vi "makeFitPlotCommands.vi"(5 "Fit Zmin":dbl=500.0 min=0.0, 6 "plotInfoArray":T1(array[cluster]), 7 "Fit Zmax":dbl=500.0 min=0.0, 9 "BL Targets":T2[](array[typedef]) {"n" min=0.02 max=0.5 step=0.01 format="%.2f"}, 10 "Coefficients":cluster{"No d0":T3, "with d0":T3}, 11 "Zref":dbl=508.0 min=0.0) -> (1 "UnderlayPlotSeries":string[](array[string])=["fitmin = 100, fitmax=550, zref=508, d=16.2, n=0.121, clippedpowerlaw(x) w line ls 1 lw 10 lc rgb \"gray25\" title 'fit with displacement'", "fitmin = 100, fitmax=550, zref=508, d=0, n=0.133, clippedpowerlaw(x) w line ls 1 lw 8 lc rgb \"gray50\" title 'zero displacement fit'", "zref=508, d=0, n=0.170, powerlaw(x) w line ls 0 lw 1 lc rgb \"gray75\" title 'target power law'"], 2 "Pre-plot Injection":string, 3 "BasicsVisible":bool[](array[boolean]))   [LabVIEW 2021]
uses:
  PowerLaw.ctl
  BLTarget.ctl
  at.ctl
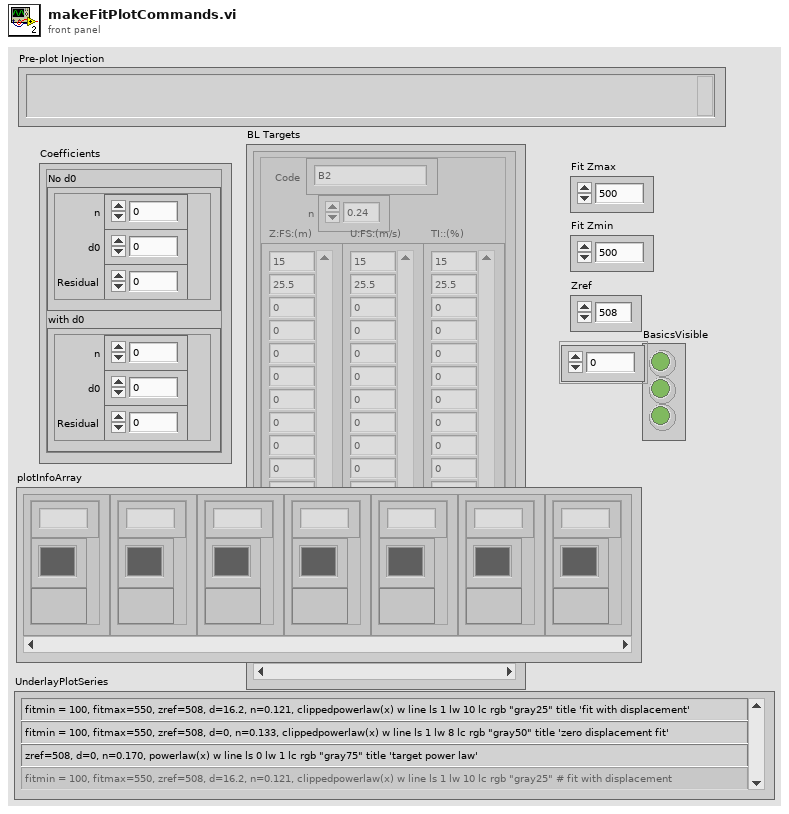
[diagram p1: front panel]
types:
  T1 = cluster{"Plot Name":string, "Plot.Plot Color":u32, "Plot.Visible?":bool}[]
  T2 = typedef "BLTarget.ctl" = cluster{"Code":string, "n":dbl, "Z:FS:(m)":dbl[], "U:FS:(m/s)":dbl[], "TI::(%)":dbl[]}
  T3 = typedef "PowerLaw.ctl" = cluster{"n":dbl, "d0":dbl, "Residual":dbl}
  T4 = typedef "at.ctl" = cluster{"XcoordSys":string, "YcoordSys":string, "Xvalue":dbl, "Yvalue":dbl}
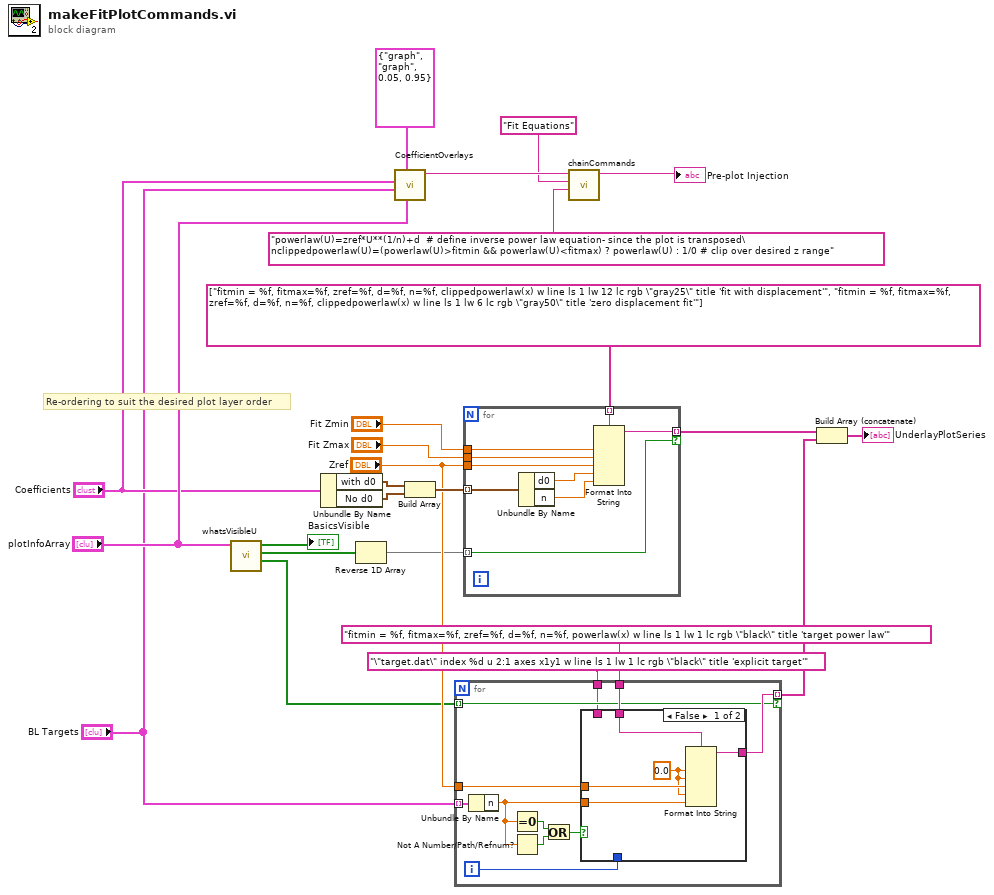
[diagram p0: block diagram]
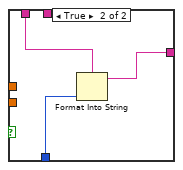
[diagram p2: hidden frame]
diagram:
  # "Re-ordering to suit the desired plot layer order"
  n1 = call "whatsVisibleU.vi"("UplotInfoArray"="plotInfoArray") -> ("Targets Visible"=w5:bool[], "Fits Visible"=w3:bool[], "BasicsVisible"=→"BasicsVisible":bool[])  [unwired: 8 in]
  n2 = Unbundle By Name("Coefficients") -> ("with d0"=w23:T3, "No d0"=w22:T3)
  n3 = Reverse 1D Array(array=w3) -> (reversed array=w4:bool[])
  n4 = call "CoefficientOverlays.vi"("plotInfoArray"="plotInfoArray", "\"At\" location"=T4 {"XcoordSys"="graph", "YcoordSys"="graph", "Xvalue"=0.05, "Yvalue"=0.95} ("\"At\" location"), "BL Targets"="BL Targets", "Coefficients"="Coefficients") -> ("gnuplotOut"=w18:string)  [unwired: 7 in]
  n5 = Build Array(w23, w22) -> (w20:T3[])
  n6 = for {
    tunnel: "fitmin = %f, fitmax=%f, zref=%f, d=%f, n=%f, powerlaw(x) w line ls 1 lw 1 lc rgb \"black\" title 'target power law'" ("String") -> [w35]
    tunnel: "BL Targets" -> [w34] mode=indexing
    tunnel: [w33] -> w9 mode=indexing if=w31
    tunnel: w5 -> [w31] mode=indexing
    tunnel: "Zref" -> [w32]
    tunnel: "\"target.dat\" index %d u 2:1 axes x1y1 w line ls 1 lw 1 lc rgb \"black\" title 'explicit target'" ("String") -> [w29]
    i -> [w30]
    n7 = Unbundle By Name(w34) -> ("n"=w28:dbl)
    n8 = Equal To 0?(x=w28) -> (x = 0?=w26:bool)
    n9 = Not A Number/Path/Refnum?(number/path/refnum=w28) -> (NaN/Path/Refnum?=w27:bool)
    n10 = Or(x=w26, y=w27) -> (x .or. y?=w25:bool)
    n11 = case shown="False" w25 {
      tunnel: w35 -> [w40 _]
      tunnel: [w39 w41] -> w33
      tunnel: w32 -> [w38 _]
      tunnel: w28 -> [w36 _]
      tunnel: w30 -> [_ w43]
      tunnel: w29 -> [_ w42]
      frame False {
        w37 = 0.0 ("input 1")
        n12 = Format Into String(format string=w40, w37, w37, w38, w37, w36) -> (resulting string=w39:string)  [unwired: 2 in, 1 out]
      }
      frame True {
        n13 = Format Into String(format string=w42, w43) -> (resulting string=w41:string)  [unwired: 2 in, 1 out]
      }
    }
  }
  n14 = for {
    tunnel: string[] ["fitmin = %f, fitmax=%f, zref=%f, d=%f, n=%f, clippedpowerlaw(x) w line ls 1 lw 12 lc rgb \"gray25\" title 'fit with displacement'", "fitmin = %f, fitmax=%f, zref=%f, d=%f, n=%f, clippedpowerlaw(x) w line ls 1 lw 6 lc rgb \"gray50\" title 'zero displacement fit'"] ("UnderlayPlotSeries 2") -> [w52] mode=indexing
    tunnel: w20 -> [w51] mode=indexing
    tunnel: "Fit Zmin" -> [w50]
    tunnel: "Fit Zmax" -> [w49]
    tunnel: [w46] -> w19 mode=indexing if=w44
    tunnel: w4 -> [w44] mode=indexing
    tunnel: "Zref" -> [w45]
    n15 = Unbundle By Name(w51) -> ("d0"=w48:dbl, "n"=w47:dbl)
    n16 = Format Into String(format string=w52, w50, w49, w45, w48, w47) -> (resulting string=w46:string)  [unwired: 2 in, 1 out]
  }
  n17 = call "chainCommands.vi"("Command"="powerlaw(U)=zref*U**(1/n)+d  # define inverse power law equation- since the plot is transposed\nclippedpowerlaw(U)=(powerlaw(U)>fitmin && powerlaw(U)<fitmax) ? powerlaw(U) : 1/0 # clip over desired z range" ("FitEquations"), "Comments"="Fit Equations", "StringIn"=w18) -> ("StringOut"=→"Pre-plot Injection":string)  [unwired: 8 in]
  n18 = Build Array (concatenate)(w19, w9) -> (→"UnderlayPlotSeries":string[])
